vi "Histogram Initialization VI.vi"(8 "error in (no error)":errorcluster, 10 "Custom XML":string, 11 "Device Item Ref in":T1 format="%.0x") -> (0 "error out":errorcluster, 3 "Device Item Ref out":T1 format="%.0x")   [LabVIEW 2012, in "Histogram Custom Device.lvlib"]
uses:
  Histogram Custom Device.lvlib
  <vilib>/NI Veristand/Custom Device API/Custom Device API.lvlib
  <vilib>/NI Veristand/Custom Device API/Custom Device Channel Type.ctl
  <vilib>/NI Veristand/Custom Device API/Custom Device Channel.ctl
  BinBounds.ctl
  <vilib>/NI Veristand/Custom Device API/Set Item Property (Variant).vi
  <vilib>/NI Veristand/Custom Device API/Custom Device Item Ref.ctl
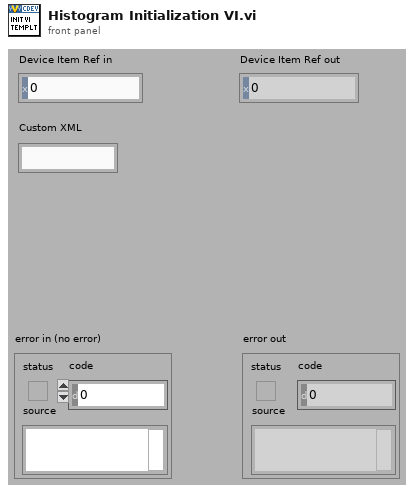
[diagram p1: front panel]
types:
  T1 = typedef "Custom Device API.lvlib/Custom Device Item Ref.ctl" = u64
  T2 = typedef "Histogram Custom Device.lvlib/BinBounds.ctl" = cluster{"Bin Counts":i32[], "Upper Bounds":dbl[], "Lower Bounds":dbl[]}
  T3 = typedef "Custom Device API.lvlib/Custom Device Channel.ctl" = cluster{"Type":T4, "Units":string, "Default Value":dbl, "Faultable":bool, "Scalable":bool}
  T4 = typedef "Custom Device API.lvlib/Custom Device Channel Type.ctl" = enum16{"Input", "Output"}
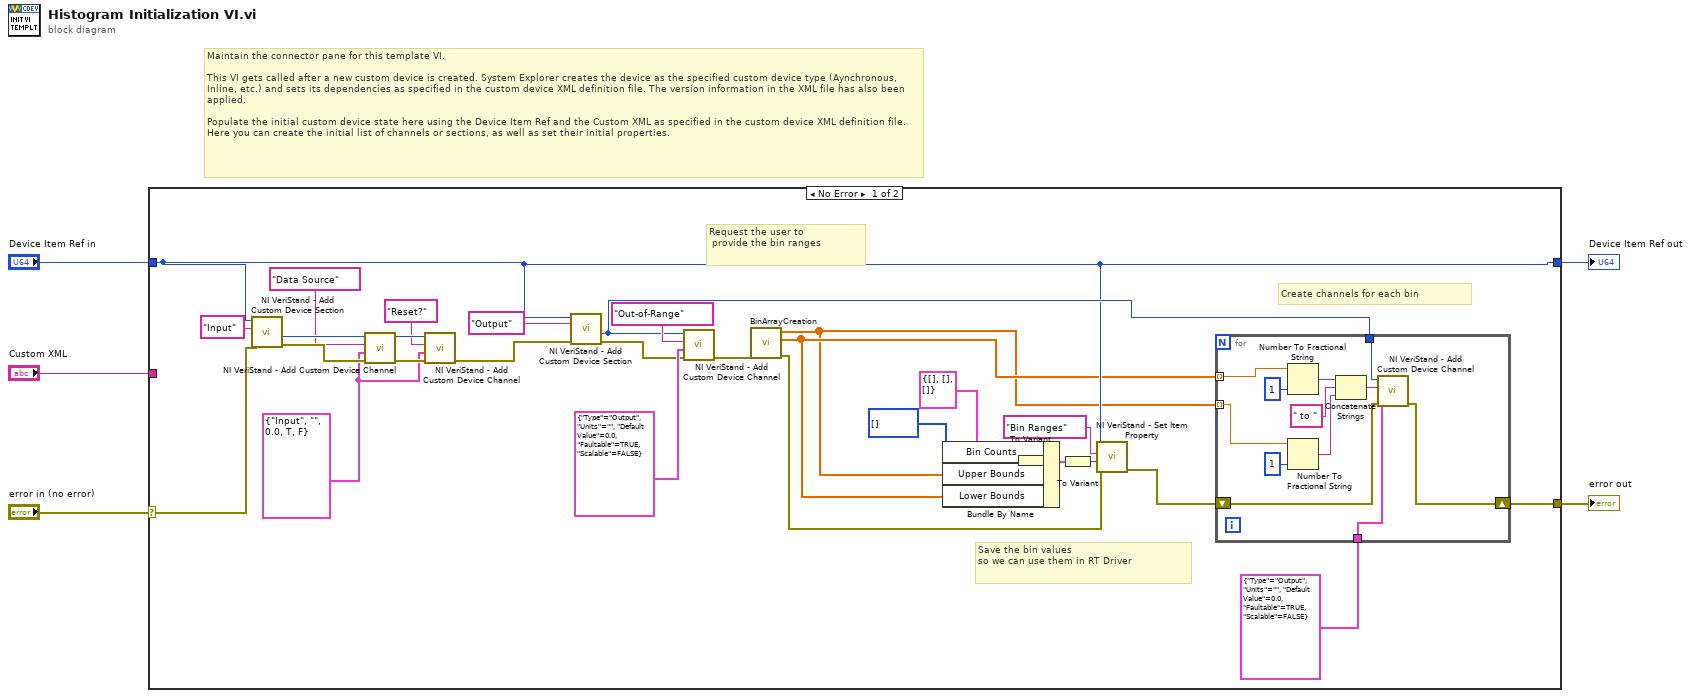
[diagram p0: block diagram]
diagram:
  # "Maintain the connector pane for this template VI.\n\nThis VI gets called after a new custom device is created. System Explorer creates the device as the specified custom device type (Aynchronous, Inline, etc.) and sets its dependencies as specified in the custom device XML definition file. The version information in the XML file has also been applied.\n\nPopulate the initial custom device state here using the Device Item Ref and the Custom XML as specified in the custom device XML definition file. Here you can create the initial list of channels or sections, as well as set their initial properties."
  n1 = case shown="No Error" "error in (no error)" {
    selector: "error in (no error)" -> [w33 w47]
    tunnel: [w22 w47] -> w5
    tunnel: [w20 w46] -> w3
    tunnel: "Device Item Ref in" -> [w20 w46]
    tunnel: "Custom XML" -> [_ _]
    frame No Error {
      w13 = T3 {"Type"=enum."Input", "Units"="", "Default Value"=0.0, "Faultable"=TRUE, "Scalable"=FALSE} ("Channel")
      # "Request the user to\n provide the bin ranges"
      # "Create channels for each bin"
      # "Save the bin values\nso we can use them in RT Driver"
      n2 = call <vilib>:"NI VeriStand - Add Custom Device Section.vi"("error in (no error)"=w33, "Section Name"="Input", "Parent Ref in"=w20) -> ("error out"=w31:errorcluster, "Section Ptr"=w30:T1)  [unwired: 5 in, 2 out]
      n3 = call <vilib>:"NI VeriStand - Add Custom Device Channel.vi"("error in (no error)"=w31, "Channel"=w13, "Channel Name"="Data Source", "Parent Ref in"=w30) -> ("error out"=w24:errorcluster, "Parent Ref out"=w14:T1)  [unwired: 4 in, 2 out]
      n4 = call <vilib>:"NI VeriStand - Add Custom Device Channel.vi"("error in (no error)"=w24, "Channel"=w13, "Channel Name"="Reset?", "Parent Ref in"=w14) -> ("error out"=w15:errorcluster)  [unwired: 4 in, 3 out]
      n5 = call <vilib>:"NI VeriStand - Add Custom Device Section.vi"("error in (no error)"=w15, "Section Name"="Output", "Parent Ref in"=w20) -> ("error out"=w26:errorcluster, "Section Ptr"=w21:T1)  [unwired: 5 in, 2 out]
      n6 = call <vilib>:"NI VeriStand - Add Custom Device Channel.vi"("error in (no error)"=w26, "Channel"=T3 {"Type"=enum."Output", "Units"="", "Default Value"=0.0, "Faultable"=TRUE, "Scalable"=FALSE}, "Channel Name"="Out-of-Range", "Parent Ref in"=w21) -> ("error out"=w11:errorcluster)  [unwired: 4 in, 3 out]
      n7 = call "BinArrayCreation.vi"("error in (no error)"=w11) -> ("error out"=w8:errorcluster, "Lower Bounds"=w10:dbl[], "Upper Bounds"=w9:dbl[])  [unwired: 8 in]
      n8 = Bundle By Name(cluster=T2 {"Bin Counts"=[], "Upper Bounds"=[], "Lower Bounds"=[]} ("Cluster"), "Bin Counts"=i32[] [], "Upper Bounds"=w9, "Lower Bounds"=w10) -> (w7:T2)
      n9 = To Variant(anything=w7) -> ()  [unwired: 1 out]
      n10 = To Variant(anything=w7) -> (Variant=w6:variant)
      n11 = call-poly <vilib>:"NI VeriStand - Set Item Property.vi"("error in (no error)"=w8, "Value"=w6, "Property Name"="Bin Ranges", "Item Ref in"=w20) -> ("error out"=w18:errorcluster)  [unwired: 5 in, 2 out]
      n12 = for {
        tunnel: T3 {"Type"=enum."Output", "Units"="", "Default Value"=0.0, "Faultable"=TRUE, "Scalable"=FALSE} ("Channel") -> [w45]
        shift-right: [w39] -> w22
        shift-left: w18 -> [w44]
        tunnel: w21 -> [w38]
        tunnel: w9 -> [w35] mode=indexing
        tunnel: w10 -> [w34] mode=indexing
        n13 = Number To Fractional String(number=w34, precision (6)=i16 1) -> (F-format string=w43:string)  [unwired: 2 in]
        n14 = Number To Fractional String(number=w35, precision (6)=i16 1) -> (F-format string=w42:string)  [unwired: 2 in]
        n15 = Concatenate Strings(w43, " to " ("string"), w42) -> (w40:string)
        n16 = call <vilib>:"NI VeriStand - Add Custom Device Channel.vi"("error in (no error)"=w44, "Channel"=w45, "Channel Name"=w40, "Parent Ref in"=w38) -> ("error out"=w39:errorcluster)  [unwired: 4 in, 3 out]
      }
    }
    frame Error {
    }
  }
  "error out" <- w5
  "Device Item Ref out" <- w3
